vi "Find Pupil2.vi"(7 "error in":errorcluster) -> (27 "error out":errorcluster)   [LabVIEW 2014]
uses:
  <vilib>/vision/Measure.llb/Edge Options.ctl
  <vilib>/vision/Measure.llb/Edge Polarity.ctl
  <vilib>/vision/NI_Vision_Development_Module.lvlib
panel:
  out "Image Out":T1(plugin-control)
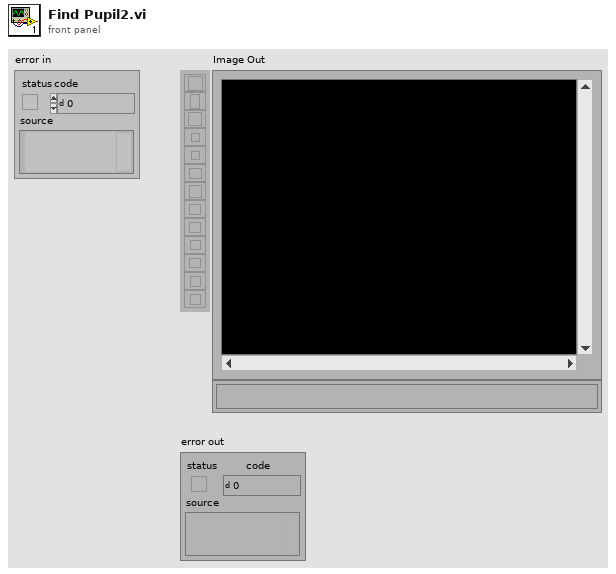
[diagram p1: front panel]
types:
  T1 = typedef "IMAQ Image.ctl" = refnum<image>
  T2 = typedef "Edge Options.ctl" = cluster{"Edge Polarity":T3, "Kernel Size":u32, "Width":u32, "Minimum Edge Strength":sgl, "Interpolation Type":enum32{"Zero Order", "Bilinear", "Quadratic", "Cubic", "Bilinear Fixed"}, "Data Processing Method":enum32{"Average", "Median"}}
  T3 = typedef "Edge Polarity.ctl" = u32
  T4 = cluster{"Search  Direction":u32, "Edge Options":T2, "Show Search Area":bool, "Show Search Lines":bool, "Show Edges Found":bool, "Show Result":bool, "Search Area Color":u32, "Search Lines Color":u32, "Edge Locations Color":u32, "Result Color":u32, "Overlay Group Name":string}
  T5 = cluster{"Process":enum16{"Get First Edge", "Get First + Last Edge", "Get All Edges", "Get Best Edge"}, "Step Size":i32, "Max Pixel Radius":i32}
  T6 = cluster{"Global Rectangle":i32[], "Contours":cluster{"ID":enum32{"External", "Internal"}, "Type":u32, "Coordinates":i32[]}[]}
  T7 = enum32{"AutoM", "Close", "Dilate", "Erode", "Gradient", "Gradient out", "Gradient in", "Hit miss", "Open", "PClose", "POpen", "Thick", "Thin"}
  T8 = typedef "Image Type" = u32
  T9 = cluster{"histogram":u32[], "Minimal Value":sgl, "Maximal Value":sgl, "Starting Value":sgl, "Interval Width":sgl, "Mean Value":sgl, "Standard  Variation":sgl, "Area (pixels)":i32}
  T10 = cluster{"Center (Pixels)":cluster{"X":sgl, "Y":sgl}, "Radius (Pixels)":dbl, "Center (Real-World)":cluster{"X":sgl, "Y":sgl}, "Radius (Real-World)":dbl, "Roundness (Real-World)":dbl, "Average Strength":dbl, "Average SNR (dB)":dbl}
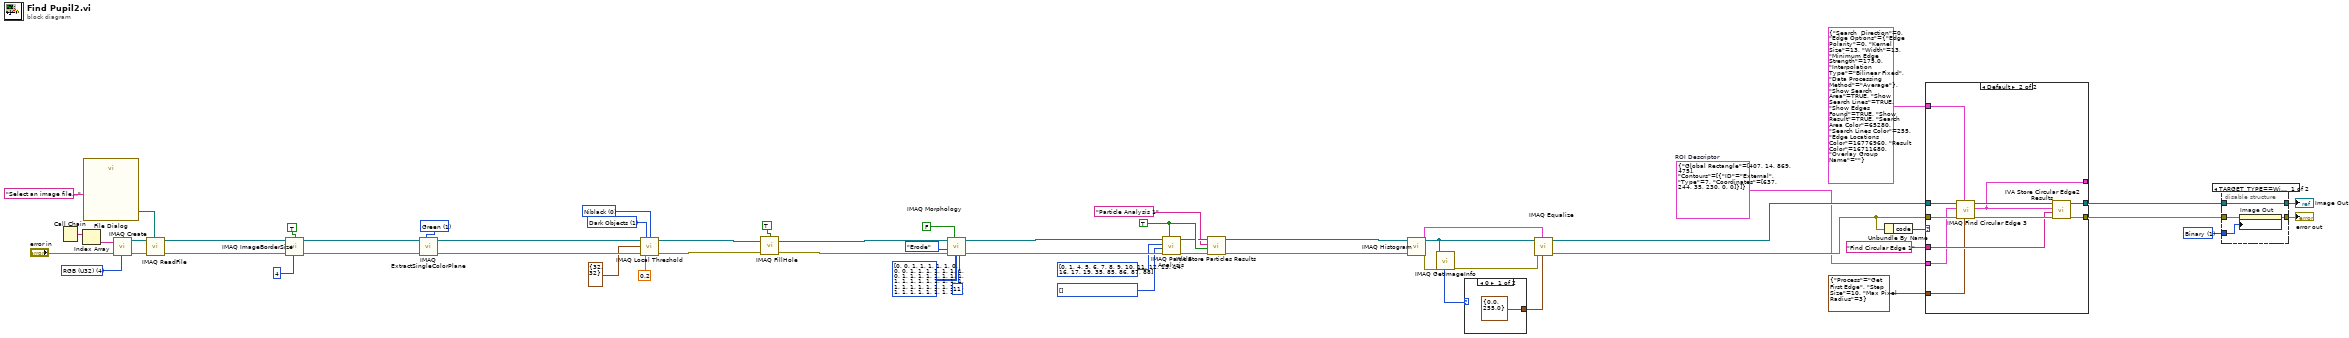
[diagram p0: block diagram]
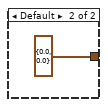
[diagram p4: hidden frame]
diagram:
  w1 = u32 1 items=["Grayscale", "Binary", "Gradient", "Rainbow", "Temperature", "User Defined"] ("Palette")
  w8 = T6 {"Global Rectangle"=[407, 14, 869, 475], "Contours"=[{"ID"=enum."External", "Type"=7, "Coordinates"=[637, 244, 35, 230, 0, 0]}]}  # ROI Descriptor
  w25 = i32[] [] items=["Center of Mass X", "Center of Mass Y", "First Pixel X", "First Pixel Y", "Bounding Rect Left", "Bounding Rect Top", "Bounding Rect Right", "Bounding Rect Bottom", "Max Feret Diameter Start X", "Max Feret Diameter Start Y", "Max Feret Diameter End X", "Max Feret Diameter End Y", "Max Horiz. Segment Length Left", "Max Horiz. Segment Length Right", "Max Horiz. Segment Length Row", "-", "Bounding Rect Width", "Bounding Rect Height", "Bounding Rect Diagonal", "Perimeter", "Convex Hull Perimeter", "Holes' Perimeter", "Max Feret Diameter", "Equivalent Ellipse Major Axis", "Equivalent Ellipse Minor Axis", "Equivalent Ellipse Minor Axis (Feret)", "Equivalent Rect Long Side", "Equivalent Rect Short Side", "Equivalent Rect Diagonal", "Equivalent Rect Short Side (Feret)", "Average Horiz. Segment Length", "Average Vert. Segment Length", "Hydraulic Radius", "Waddel Disk Diameter", "-", "Area", "Holes' Area", "Particle & Holes' Area", "Convex Hull Area", "Image Area", "-", "Number of Holes", "Number of Horiz. Segments", "Number of Vert. Segments", "-", "Orientation", "Max Feret Diameter Orientation", "-", "% Area/Image Area", "% Area/(Particle & Holes' Area)", "Ratio of Equivalent Ellipse Axes", "Ratio of Equivalent Rect Sides", "-", "Elongation Factor", "Compactness Factor", "Heywood Circularity Factor", "Type Factor", "-", "Sum X", "Sum Y", "Sum XX", "Sum XY", "Sum YY", "Sum XXX", "Sum XXY", "Sum XYY", "Sum YYY", "-", "Moment of Inertia XX", "Moment of Inertia XY", "Moment of Inertia YY", "Moment of Inertia XXX", "Moment of Inertia XXY", "Moment of Inertia XYY", "Moment of Inertia YYY", "Norm. Moment of Inertia XX", "Norm. Moment of Inertia XY", "Norm. Moment of Inertia YY", "Norm. Moment of Inertia XXX", "Norm. Moment of Inertia XXY", "Norm. Moment of Inertia XYY", "Norm. Moment of Inertia YYY", "Hu Moment 1", "Hu Moment 2", "Hu Moment 3", "Hu Moment 4", "Hu Moment 5", "Hu Moment 6", "Hu Moment 7"] ("Real-World Measurements")
  w26 = i32[] [0, 1, 4, 5, 6, 7, 8, 9, 10, 11, 12, 13, 14, 16, 17, 19, 35, 85, 86, 87, 88] items=["Center of Mass X", "Center of Mass Y", "First Pixel X", "First Pixel Y", "Bounding Rect Left", "Bounding Rect Top", "Bounding Rect Right", "Bounding Rect Bottom", "Max Feret Diameter Start X", "Max Feret Diameter Start Y", "Max Feret Diameter End X", "Max Feret Diameter End Y", "Max Horiz. Segment Length Left", "Max Horiz. Segment Length Right", "Max Horiz. Segment Length Row", "-", "Bounding Rect Width", "Bounding Rect Height", "Bounding Rect Diagonal", "Perimeter", "Convex Hull Perimeter", "Holes' Perimeter", "Max Feret Diameter", "Equivalent Ellipse Major Axis", "Equivalent Ellipse Minor Axis", "Equivalent Ellipse Minor Axis (Feret)", "Equivalent Rect Long Side", "Equivalent Rect Short Side", "Equivalent Rect Diagonal", "Equivalent Rect Short Side (Feret)", "Average Horiz. Segment Length", "Average Vert. Segment Length", "Hydraulic Radius", "Waddel Disk Diameter", "-", "Area", "Holes' Area", "Particle & Holes' Area", "Convex Hull Area", "Image Area", "-", "Number of Holes", "Number of Horiz. Segments", "Number of Vert. Segments", "-", "Orientation", "Max Feret Diameter Orientation", "-", "% Area/Image Area", "% Area/(Particle & Holes' Area)", "Ratio of Equivalent Ellipse Axes", "Ratio of Equivalent Rect Sides", "-", "Elongation Factor", "Compactness Factor", "Heywood Circularity Factor", "Type Factor", "-", "Sum X", "Sum Y", "Sum XX", "Sum XY", "Sum YY", "Sum XXX", "Sum XXY", "Sum XYY", "Sum YYY", "-", "Moment of Inertia XX", "Moment of Inertia XY", "Moment of Inertia YY", "Moment of Inertia XXX", "Moment of Inertia XXY", "Moment of Inertia XYY", "Moment of Inertia YYY", "Norm. Moment of Inertia XX", "Norm. Moment of Inertia XY", "Norm. Moment of Inertia YY", "Norm. Moment of Inertia XXX", "Norm. Moment of Inertia XXY", "Norm. Moment of Inertia XYY", "Norm. Moment of Inertia YYY", "Hu Moment 1", "Hu Moment 2", "Hu Moment 3", "Hu Moment 4", "Hu Moment 5", "Hu Moment 6", "Hu Moment 7"] ("Pixel Measurements")
  w23 = TRUE ("Connectivity 4/8 (8)")
  w37 = u32 1 items=["Bright Objects", "Dark Objects"] ("Look For (Bright Objects)")
  w40 = u32 0 items=["Niblack", "Background Correction"] ("Method")
  w44 = 1 items=["Red", "Green", "Blue", "Hue", "Saturation", "Luminance", "Value", "Intensity"] ("Color Plane")
  w49 = T8 4 items=["Grayscale (U8)", "Grayscale (I16)", "Grayscale (SGL)", "Complex (CSG)", "RGB (U32)", "HSL (U32)", "RGB (U64)", "Grayscale (U16)"] ("Image Type")
  n1 = Call Chain() -> (call chain=w53:string[])
  n2 = Index Array(array=w53) -> (element=w52:string)  [unwired: 1 in]
  n3 = call "File Dialog"("prompt"="Select an image file...") -> ("selected path"=w50:path)  [unwired: 6 in, 8 out]
  n4 = call "IMAQ Create"("Image Name"=w52, "Image Type"=w49, "error in (no error)"="error in") -> ("New Image"=w56:T1, "error out"=w55:errorcluster)  [unwired: 1 in, 1 out]
  n5 = call "IMAQ ReadFile"("File Path"=w50, "error in (no error)"=w55, "Image"=w56) -> ("error out"=w57:errorcluster, "Image Out"=w48:T1)  [unwired: 2 in, 5 out]
  n6 = call "IMAQ ImageBorderSize"("Get/Set Status? (Set)"=TRUE, "Image"=w48, "Image border size in"=4 ("Border Size"), "error in (no error)"=w57) -> ("Image Out"=w43:T1, "error out"=w47:errorcluster)  [unwired: 1 out]
  n7 = call "IMAQ ExtractSingleColorPlane"("Color Plane"=w44, "error in (no error)"=w47, "Image Src"=w43) -> ("error out"=w42:errorcluster, "Image Dst Out"=w41:T1)  [unwired: 1 in, 6 out]
  n8 = call "IMAQ Local Threshold"("Image Src"=w41, "Look For (Bright Objects)"=w37, "Method (Niblack)"=w40, "Window Size (32x32)"=cluster{"SizeX":i32, "SizeY":i32} {"SizeX"=32, "SizeY"=32} ("Kernel Size"), "error in (no error)"=w42, "Niblack Deviation Factor (0.2)"=0.2 ("Niblack Deviation Factor")) -> ("Image Dst Out"=w34:T1, "error out"=w36:errorcluster)  [unwired: 2 in, 6 out]
  n9 = call "IMAQ FillHole"("error in (no error)"=w36, "Image Src"=w34, "Connectivity 4/8 (8)"=TRUE) -> ("error out"=w33:errorcluster, "Image Dst Out"=w28:T1)  [unwired: 1 in, 2 out]
  n10 = call "IMAQ Morphology"("Number of iterations (1)"=11, "Structuring Element"=i32[][] [[0, 0, 1, 1, 1, 1, 1, 0, 0], [0, 1, 1, 1, 1, 1, 1, 1, 0], [1, 1, 1, 1, 1, 1, 1, 1, 1], [1, 1, 1, 1, 1, 1, 1, 1, 1], [1, 1, 1, 1, 1, 1, 1, 1, 1], [1, 1, 1, 1, 1, 1, 1, 1, 1], [1, 1, 1, 1, 1, 1, 1, 1, 1], [0, 1, 1, 1, 1, 1, 1, 1, 0], [0, 0, 1, 1, 1, 1, 1, 0, 0]], "Square/Hexa (Square)"=FALSE, "error in (no error)"=w33, "Operation"=T7."Erode", "Image Src"=w28) -> ("error out"=w27:errorcluster, "Image Dst Out"=w24:T1)  [unwired: 1 in, 3 out]
  n11 = call "IMAQ Particle Analysis"("Connectivity 4/8 (8)"=w23, "error in (no error)"=w27, "Real-World Measurements"=w25, "Pixel Measurements"=w26, "Image"=w24) -> ("error out"=w20:errorcluster, "Image Out (duplicate)"=w22:T1)  [unwired: 5 out]
  n12 = call <vilib>:"IVA Store Particles Results.vi"("error in (no error)"=w20, "Connectivity 4/8 (8)"=w23, "Step Name"="Particle Analysis 1", "Image in"=w22) -> ("error out"=w19:errorcluster, "Image dup"=w15:T1)  [unwired: 6 out]
  n13 = call "IMAQ Histogram"("error in (no error)"=w19, "Image"=w15) -> ("error out"=w14:errorcluster, "Histogram Report"=w17:T9)  [unwired: 3 in, 5 out]
  n14 = call "IMAQ GetImageInfo"("error in (no error)"=w14, "Image"=w15) -> ("error out"=w13:errorcluster, "Image Type"=w16:T8)  [unwired: 8 out]
  n15 = case shown="0" w16 {
    tunnel: [cluster{"Minimum":sgl, "Maximum":sgl} {"Minimum"=0.0, "Maximum"=255.0} ("Range") cluster{"Minimum":sgl, "Maximum":sgl} {"Minimum"=0.0, "Maximum"=0.0} ("Range")] -> w12
    frame 0 {
    }
    frame Default {
    }
  }
  n16 = call "IMAQ Equalize"("Range"=w12, "Histogram Report"=w17, "error in (no error)"=w13, "Image Src"=w15) -> ("error out"=w18:errorcluster, "Image Dst Out"=w11:T1)  [unwired: 2 in, 4 out]
  n17 = Unbundle By Name(w18) -> ("code"=w7:i32)
  n18 = case shown="Default" w7 {
    tunnel: T4 {"Search  Direction"=0, "Edge Options"={"Edge Polarity"=0, "Kernel Size"=13, "Width"=13, "Minimum Edge Strength"=175.0, "Interpolation Type"=enum."Bilinear Fixed", "Data Processing Method"=enum."Average"}, "Show Search Area"=TRUE, "Show Search Lines"=TRUE, "Show Edges Found"=TRUE, "Show Result"=TRUE, "Search Area Color"=65280, "Search Lines Color"=255, "Edge Locations Color"=16776960, "Result Color"=16711680, "Overlay Group Name"=""} ("Options") -> [_ w61]
    tunnel: w11 -> [w60 w71]
    tunnel: w18 -> [_ w70]
    tunnel: [_ w68] -> w10
    tunnel: [w60 w66] -> w3
    tunnel: "Find Circular Edge 1" ("Step Name") -> [_ w65]
    tunnel: w8 -> [_ w64]
    tunnel: T5 {"Process"=enum."Get First Edge", "Step Size"=10, "Max Pixel Radius"=3} ("Circle Fit Options") -> [_ w63]
    tunnel: [_ w62] -> _
    frame -1074396199, -1074396198 {
      # "Discard Coordinate System Error"
    }
    frame Default {
      n19 = call "IMAQ Find Circular Edge 3"("Circle Fit Options"=w63, "Options"=w61, "error in (no error)"=w70, "ROI Descriptor"=w64, "Image"=w71) -> ("error out"=w69:errorcluster, "Fitted Circle"=w62:T10, "Image Out"=w67:T1)  [unwired: 2 in, 2 out]
      n20 = call <vilib>:"IVA Store Circular Edge2 Results.vi"("error in (no error)"=w69, "Step Name"=w65, "Fitted Circle"=w62, "Image in"=w67) -> ("error out"=w68:errorcluster, "Image dup"=w66:T1)  [unwired: 2 in, 4 out]
    }
  }
  n21 = disable-structure "Conditional Disable Structure" shown="TARGET_TYPE==Windows" {
    disable-tunnel: w10 -> [w75 w76]
    disable-tunnel: [w74 w76] -> w4
    disable-tunnel: w3 -> [w73 w77]
    disable-tunnel: [w73 w77] -> w2
    disable-tunnel: w1 -> [w72 _]
    frame condition #0 (active) {
      n22 = property on="Image Out" class="ImageControl"(error in=w75, "Palette:Palette Type"=w72) -> (error out=w74:errorcluster)  [unwired: 1 in, 1 out]
    }
    frame condition #1 {
    }
  }
  "error out" <- w4
  "Image Out" <- w2
